vi "Conditional State String.vi"(7 "Do State(s)?":bool, 8 "State":string) -> (5 "State Out":string)   [LabVIEW 2020]
doc: "Conditionally passes the <b>State</b> string though the function when <b>Do State(s)?</b> is TRUE.\n\nFor instructions on how to use the JKI State Machine, examples and video tutorials, visit:\nhttp://jkisoft.com/state-machine/"
panel:
  # "For instructions on how to use the JKI State Machine, examples and video tutorials, visit:\nhttp://jki.net/state-machine/\n\nJKI State Machine™\nhttp://jki.net/state-machine/\nCopyright (C) 2005-2024, JKI <info@jki.net>\nALL RIGHTS RESERVED"
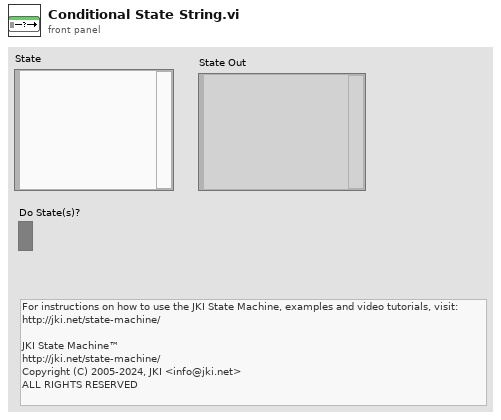
[diagram p1: front panel]
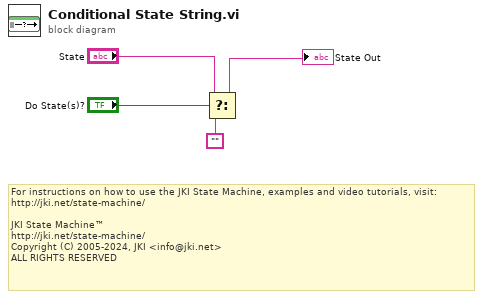
[diagram p0: block diagram]
diagram:
  # "For instructions on how to use the JKI State Machine, examples and video tutorials, visit:\nhttp://jki.net/state-machine/\n\nJKI State Machine™\nhttp://jki.net/state-machine/\nCopyright (C) 2005-2024, JKI <info@jki.net>\nALL RIGHTS RESERVED"
  n1 = Select(t="State", s="Do State(s)?", f="") -> (s? t:f=→"State Out":string)
